vi "oax_Update Cursor Position.vi"(8 "speed profile":T1 {"speed [RPM]" format="%.2f"; "time [s]" format="%.2f"}, 9 "Order to preview":dbl=1.0 min=0.01 format="%#.2g", 11 "Cursor Position":cluster{"X":dbl, "Y":dbl}) -> (3 "Cursor Position Out":cluster{"time [s]":dbl, dbl})   [LabVIEW 2017]
uses:
  <vilib>/addons/Sound and Vibration/Order Analysis/Tach Process/SubVIs/speed profile.ctl
  <vilib>/addons/Sound and Vibration/Order Analysis/Tach Process/SoundVib_TachProcess.lvlib
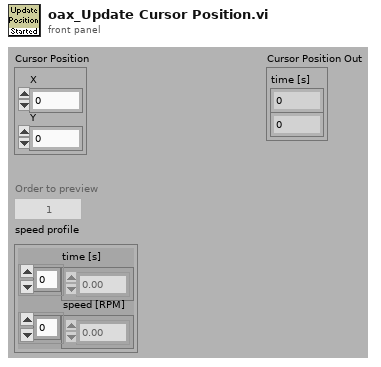
[diagram p1: front panel]
types:
  T1 = typedef "SoundVib_TachProcess.lvlib/speed profile.ctl" = cluster{"time [s]":dbl[], "speed [RPM]":dbl[]}
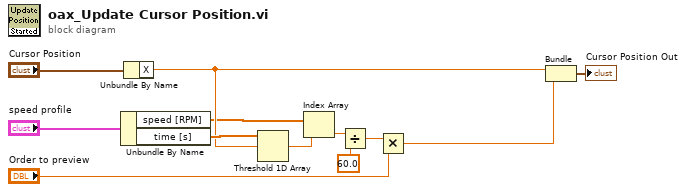
[diagram p0: block diagram]
diagram:
  n1 = Unbundle By Name("speed profile") -> ("speed [RPM]"=w7:dbl[], "time [s]"=w10:dbl[])
  n2 = Unbundle By Name("Cursor Position") -> ("X"=w9:dbl)
  n3 = Threshold 1D Array(2:w9, 3:w10) -> (0:w8:dbl)  [unwired: 1 in]
  n4 = Index Array(array=w7, index=w8) -> (element=w2:dbl)
  n5 = Divide(x=w2, y=60.0 ("x")) -> (x/y=w6:dbl)
  n6 = Multiply(x=w6, y="Order to preview") -> (x*y=w4:dbl)
  n7 = Bundle("X"=w9, w4) -> (→"Cursor Position Out":cluster{"X":dbl, dbl})  [unwired: 1 in]
